vi "UA_XML_Read.vi"(8 "error in (no error)":errorcluster caption="错误输入（无错误）", 11 "XML File Path":path=path "E:/快盘/兰州项目资料/OPCUA XML_8.19/RT/test.xml") -> (0 "error out":errorcluster caption="错误输出", 2 "xml Data":string[](array[string]), 3 "XML File Path":path=path "C:/Users/isleep/Desktop/OPCUA XML/RT/test.xml")   [LabVIEW 2013, in "OPCUA XML.lvlib"]
uses:
  OPCUA XML.lvlib
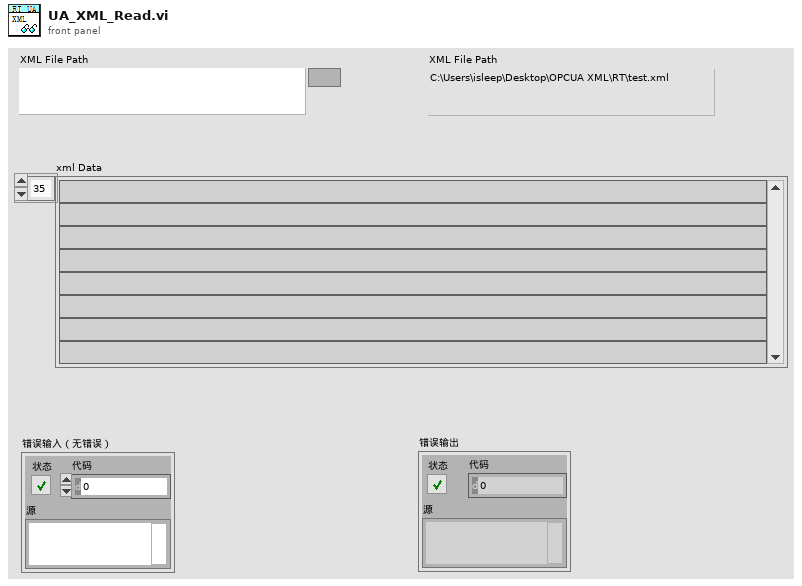
[diagram p1: front panel]
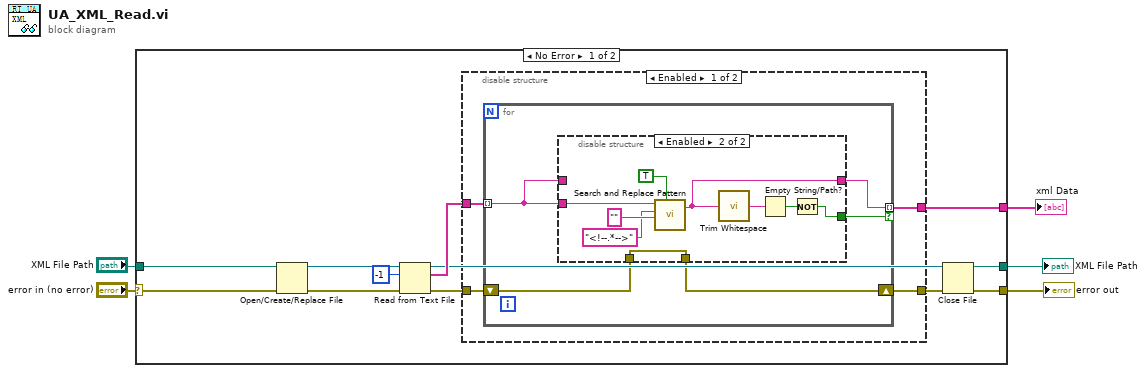
[diagram p0: block diagram]
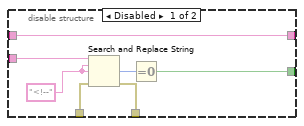
[diagram p2: hidden frame]
diagram:
  n1 = case shown="No Error" "error in (no error)" {
    selector: "error in (no error)" -> [w12 w46]
    tunnel: [w11 w46] -> w4
    tunnel: "XML File Path" -> [w10 w45]
    tunnel: [w7 w45] -> w2
    tunnel: [w6 _] -> w1
    frame No Error {
      n2 = Open/Create/Replace File(file path (use dialog)=w10, error in=w12) -> (refnum out=w17:refnum<file>, error out=w14:errorcluster)  [unwired: 4 in, 1 out]
      n3 = Read from Text File(file (use dialog)=w17, count=-1 ("计数"), error in=w14) -> (refnum out=w13:refnum<file>, text=w15:string[], error out=w9:errorcluster)  [unwired: 1 in, 1 out]
      n4 = disable-structure shown="Enabled" {
        disable-tunnel: w15 -> [w21 w43]
        disable-tunnel: w9 -> [w20 w44]
        disable-tunnel: [w19 w44] -> w8
        disable-tunnel: [w18 w43] -> w6
        frame Enabled {
          n5 = for {
            tunnel: w21 -> [w23] mode=indexing
            tunnel: [w24] -> w18 mode=indexing if=w22
            shift-right: [w25] -> w19
            shift-left: w20 -> [w26]
            n6 = disable-structure shown="Enabled" {
              disable-tunnel: w23 -> [w33 w39]
              disable-tunnel: w26 -> [w32 w38]
              disable-tunnel: [w31 w38] -> w25
              disable-tunnel: [w29 w37] -> w24
              disable-tunnel: w23 -> [w29 _]
              disable-tunnel: [w27 w34] -> w22
              frame Disabled {
                w30 = "<!--" ("搜索字符串/字符(-)")
                n7 = Search and Replace String(input string=w33, search string=w30, replace string=w30, error in=w32) -> (number of replacements=w28:i32, error out=w31:errorcluster)  [unwired: 4 in, 2 out]
                n8 = Equal To 0?(x=w28) -> (x = 0?=w27:bool)
              }
              frame Enabled {
                n9 = call <vilib>:"Search and Replace Pattern.vi"("string"=w39, "regular expression (\"\")"="<!--.*-->" ("regular expression (\"\")"), "replace string (\"\")"="" ("replace string (\"\")"), "replace all? (F)"=TRUE) -> ("result string"=w37:string)  [unwired: 1 in, 1 out]
                n10 = call <vilib>:"Trim Whitespace.vi"("string"=w37) -> ("trimmed string"=w35:string)  [unwired: 1 in]
                n11 = Empty String/Path?(string/path=w35) -> (empty?=w36:bool)
                n12 = Not(x=w36) -> (.not. x?=w34:bool)
              }
            }
          }
        }
        frame Disabled {
        }
      }
      n13 = Close File(refnum=w13, error in=w8) -> (path=w7:path, error out=w11:errorcluster)
    }
    frame Error {
    }
  }
  "error out" <- w4
  "XML File Path" <- w2
  "xml Data" <- w1
